vi "Settings_TestCase_NewTestCaseNumber.vi"(8 "error in":errorcluster, 11 "VI Server Cluster":T1) -> (0 "error out":errorcluster, 2 "Update?":bool, 3 "VI Server ClusterDUP":T1)   [LabVIEW 2020]
uses:
  LabVIEW 2020 Toolkits/VI Server Toolkit/VI Server Toolkit LV2013.lvlib
  Instruments/NA-E5071B/E5071B.llb/Labels&Control References.ctl
panel:
  in  "Done":bool
  in  "Cancel":bool
  in  "NewTestCase":string caption="Enter New Case Number"
  # "NOTE:\nPlease follow the Test Case numbering convention:\n1.3; 1.2; 1.3; etc."
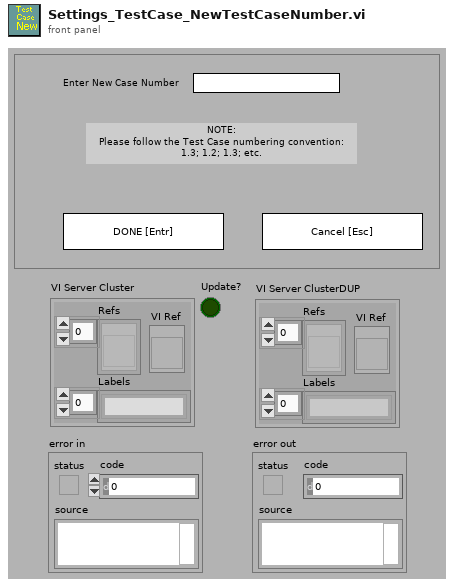
[diagram p1: front panel]
types:
  T1 = typedef "Labels&Control References.ctl" = cluster{"Refs":refnum<vi>[], "Labels":string[], "VI Ref":refnum<vi>}
  T2 = typedef "VI Server_RefsCluster.ctl" = cluster{"Labels":string[], "Refs":refnum<vi>[], "VI Ref":refnum<vi>}
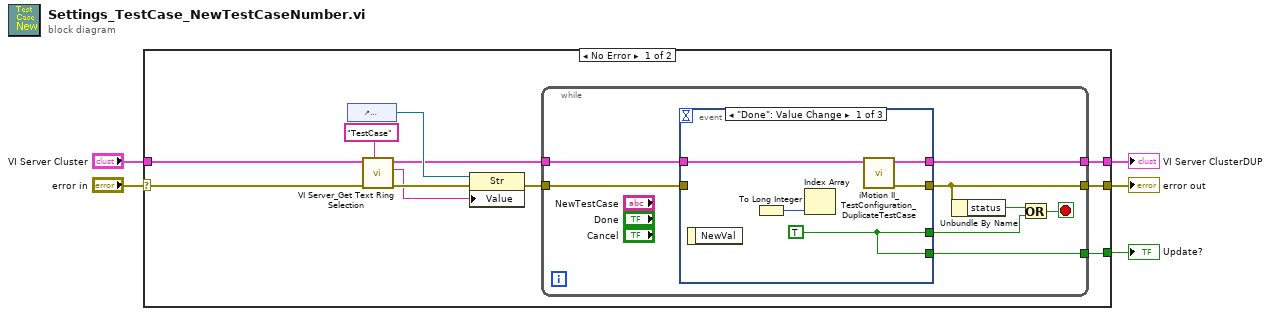
[diagram p0: block diagram]
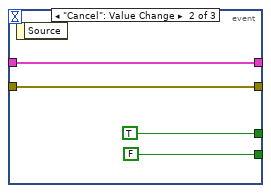
[diagram p2: hidden frame]
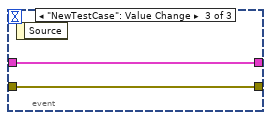
[diagram p3: hidden frame]
diagram:
  n1 = case shown="No Error" "error in" {
    selector: "error in" -> [w12 w37]
    tunnel: [w16 w37] -> w5
    tunnel: "VI Server Cluster" -> [w11 _]
    tunnel: [w14 _] -> w2
    tunnel: [w13 _] -> w1
    frame No Error {
      n2 = control-ref of="NewTestCase"() -> (w15:refnum<vi>)
      n3 = call "VI Server_Get Text Ring Selection.vi"("Label"="TestCase", "error in"=w12, "VI Server Cluster"=w11) -> ("error out"=w8:errorcluster, "Selection"=w7:string, "VI Server Custer.DUP"=w10:T2)  [unwired: 3 in, 3 out]
      n4 = property class="Str"(reference=w15, error in=w8, "Value"=w7) -> (error out=w6:errorcluster)  [unwired: 1 out]
      n5 = while {
        tunnel: [w22] -> w16
        tunnel: w6 -> [w24]
        tunnel: w10 -> [w23]
        tunnel: [w18] -> w14
        tunnel: [w17] -> w13
        stop <- w20 stop-if-true
        n6 = event shown="[0] \"Done\": Value Change" {
          selector: _ -> [_ _ _]
          dyn-events: _ -> [_ _ _]
          timeout: _ -> [_ _ _]
          tunnel: [w30 w34 w36] -> w22
          tunnel: w24 -> [_ w34 w36]
          tunnel: w23 -> [w29 w32 w35]
          tunnel: [w25 TRUE _] -> w19
          tunnel: [w26 w32 w35] -> w18
          tunnel: [w25 FALSE _] -> w17
          event "Done": Value Change {
            w25 = TRUE
            n7 = event-data() -> ()  [unwired: 1 in, 1 out]
            n8 = To Long Integer() -> (32bit integer=w27:i32)  [unwired: 1 in]
            n9 = Index Array(index=w27) -> ()  [unwired: 1 in, 1 out]
            n10 = call "iMotion II_TestConfiguration_DuplicateTestCase.vi"("Data Cluster"=w29) -> ("error out"=w30:errorcluster, "Data Cluster DUP"=w26:T1, "error in (no error)"=w28:errorcluster)  [unwired: 8 in]
          }
          event "Cancel": Value Change {
            n11 = event-data() -> ()  [unwired: 1 in, 1 out]
          }
          event "NewTestCase": Value Change {
            n12 = event-data() -> ()  [unwired: 1 in, 1 out]
          }
        }
        n13 = Unbundle By Name(w22) -> ("status"=w21:bool)
        n14 = Or(x=w21, y=w19) -> (x .or. y?=w20:bool)
      }
    }
    frame Error {
    }
  }
  "error out" <- w5
  "VI Server ClusterDUP" <- w2
  "Update?" <- w1
